vi "AddTestWithoutData.vi"(8 "error in (no error)":errorcluster, 10 "Path":path, 11 "TestSuite in":refnum<class "TestSuite.lvclass">) -> (0 "error out":errorcluster, 3 "TestSuite out":refnum<class "TestSuite.lvclass">)   [LabVIEW 2019, in "TestSuite.lvclass"]
uses:
  TestSuite.lvclass
  TestCase/Fact/Fact.lvclass
  C:/Users/de200256/Code/LVUnit/TestCase/TestCase/TestCase.lvclass
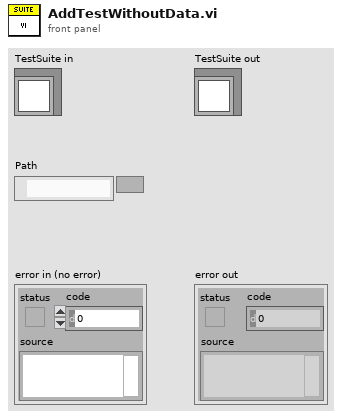
[diagram p1: front panel]
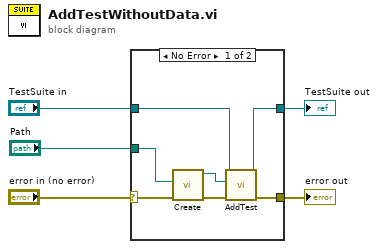
[diagram p0: block diagram]
diagram:
  n1 = case shown="No Error" "error in (no error)" {
    selector: "error in (no error)" -> [w6 w14]
    tunnel: [w11 w14] -> w4
    tunnel: [w9 w13] -> w2
    tunnel: "TestSuite in" -> [w10 w13]
    tunnel: "Path" -> [w7 _]
    frame No Error {
      n2 = call "Create.vi"("error in (no error)"=w6, "Path"=w7) -> ("error out"=w12:errorcluster, "Fact"=w8:refnum<class "Fact.lvclass">)  [unwired: 8 in]
      n3 = call-dynamic "AddTest.vi"("error in (no error)"=w12, "TestCase"=w8, "TestSuite in"=w10) -> ("error out"=w11:errorcluster, "TestSuite out"=w9:refnum<class "TestSuite.lvclass">)  [unwired: 7 in]
    }
    frame Error {
    }
  }
  "error out" <- w4
  "TestSuite out" <- w2
